vi "Get Section.vi"(11 "TypeDefinitions in":refnum<class "TypeDefinitions.lvclass">) -> (2 "Section":string, 3 "TypeDefinitions out":refnum<class "TypeDefinitions.lvclass">)   [LabVIEW 2024, in "Electronic Datasheet.lvlib" / "TypeDefinitions.lvclass"]
uses:
  TypeDefinitions.lvclass
  TypeDefinitions.lvclass/TypeDefinitions.ctl
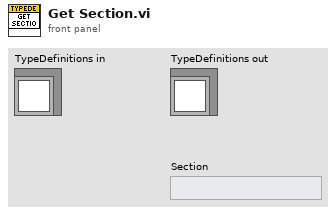
[diagram p1: front panel]
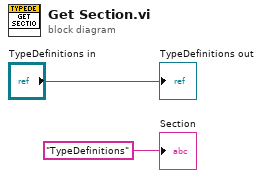
[diagram p0: block diagram]
diagram:
  "TypeDefinitions out" <- "TypeDefinitions in"
  "Section" <- "TypeDefinitions" ("Section")
